vi "Write Single Holding Register.vi"(8 "error in":errorcluster, 9 "register to write":u16, 10 "address":u16, 11 "Modbus instance in":refnum<class "Modbus API.lvclass">) -> (0 "error out":errorcluster, 3 "Modbus instance out":refnum<class "Modbus API.lvclass">)   [LabVIEW 2021, in "Modbus API.lvclass"]
doc: "Writes <B>register to write</B> to <B>address</B> of the device."
uses:
  Modbus API.lvclass
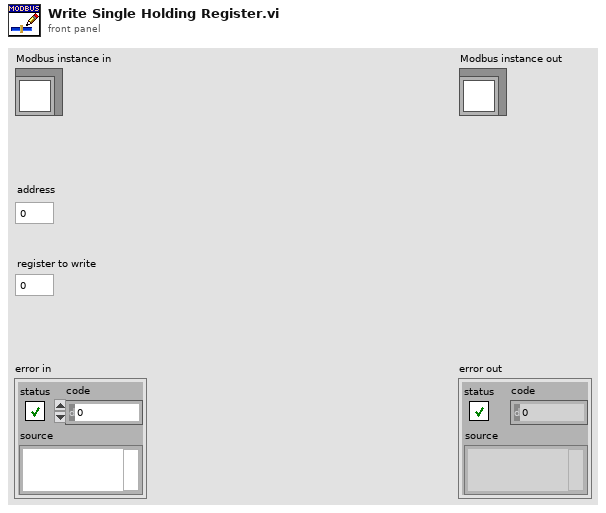
[diagram p1: front panel]
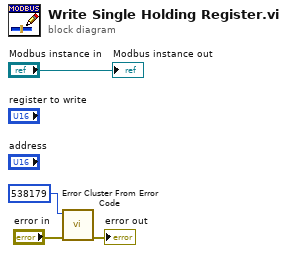
[diagram p0: block diagram]
diagram:
  n1 = call <vilib>:"Error Cluster From Error Code.vi"("error in (no error)"="error in", "error code (0)"=538179) -> ("error out"=→"error out":errorcluster)  [unwired: 7 in]
  "Modbus instance out" <- "Modbus instance in"
